vi "ReadLatchMatrix.vi"() -> ()   [LabVIEW 2014]
panel:
  in  "error in (no error)":errorcluster
  out "error out":errorcluster
  out "String 4":string
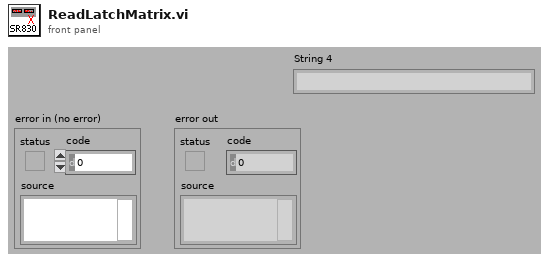
[diagram p1: front panel]
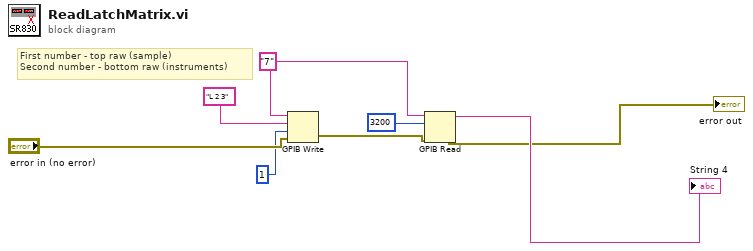
[diagram p0: block diagram]
diagram:
  w3 = "7"
  # "First number - top raw (sample)\nSecond number - bottom raw (instruments)"
  n1 = GPIB Write(0:w3, 1:"L 2 3", 2:1, 3:"error in (no error)") -> (6:w8:errorcluster)  [unwired: 1 in, 1 out]
  n2 = GPIB Read(0:w3, 1:3200, 3:w8) -> (5:→"String 4":string, 7:→"error out":errorcluster)  [unwired: 2 in, 1 out]
